vi "HP Loop.vi"(8 "error in (no error)":errorcluster, 11 "ValveControlModule in":refnum<class "ValveControlModule.lvclass">) -> (0 "error out":errorcluster, 3 "ValveControlModule out":refnum<class "ValveControlModule.lvclass">)   [LabVIEW 2020, in "VolatusControl.lvlib" / "ValveControlModule.lvclass"]
uses:
  ValveControlModule.lvclass
  ValveControlModule.lvclass/ValveControlModule.ctl
  <vilib>/Platform/TimedLoop/XDataNode/wakeup.ctl
  <vilib>/Platform/TimedLoop/XDataNode/XDNodeRunTimeDep.lvlib
  <vilib>/Platform/TimedLoop/XDataNode/nitl_modes.ctl
  <vilib>/Platform/TimedLoop/XDataNode/timing_clust.ctl
  <vilib>/platform/TimedLoop/XDataNode/XDataNode.xnode
  Volatus/Module/Module.lvclass
  messages/CmdDigital/Class/Msg.lvclass
  messages/CmdDigital/Data.ctl
  messages/CmdDigital/CmdDigital.lvlib
  messages/CmdDigitalMultiple/Data.ctl
  messages/CmdDigitalMultiple/CmdDigitalMultiple.lvlib
  messages/CmdAnalog/Class/Msg.lvclass
  messages/CmdAnalog/Data.ctl
  messages/CmdAnalog/CmdAnalog.lvlib
  lv-vecto/Vecto/GroupAbstract/GroupAbstract.lvclass
  C:/dev/lv20CE/relink/lv-volatus/Volatus/Module/Module.lvclass
  C:/dev/lv20CE/relink/lv-volatus/VolatusControl/ValveControlModule/ValveControlModule.lvclass
  C:/dev/lv20CE/relink/lv-volatus/messages/CmdDigital/Class/Msg.lvclass
  C:/dev/lv20CE/relink/lv-protoc/LV-Proto/Message/Message.lvclass
  C:/dev/lv20CE/relink/lv-volatus/messages/CmdAnalog/Class/Msg.lvclass
  lv-vecto/Vecto/Group/Group.lvclass
  C:/dev/lv20CE/relink/lv-vecto/Vecto/GroupAbstract/GroupAbstract.lvclass
  C:/dev/lv20CE/relink/lv-vecto/Vecto/Group/Group.lvclass
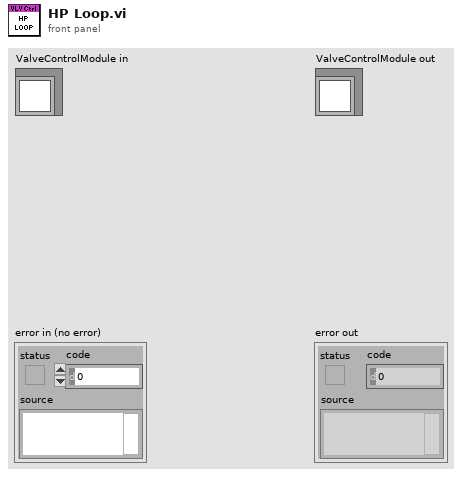
[diagram p1: front panel]
types:
  T1 = typedef "XDNodeRunTimeDep.lvlib/timing_clust.ctl" = cluster{"Expected End [f-1]":u64, "Actual End [f-1]":u64, "Finished Late? [f-1]":bool, "Expected End [i-1]":u64, "Actual End [i-1]":u64, "Finished Late? [i-1]":bool, "Expected Start [i]":u64, "Actual Start [i]":u64, "Expected Start [f]":u64, "Actual Start [f]":u64, "Source Name":string, "Structure Name":string, "Period":i64, "Deadline":i64, "Offset":i64, "Start":i64, "Priority":i32, "Timeout":i32, "Mode":T2, "Wakeup Reason":T3, "Error":errorcluster, "Source Type":string, "Secondary Source Type":string, "Global End Time":u64, "Global Start Time":u64, "Frame Duration":u64, "Iteration Duration":u64, "Assigned CPU":i32, "I/O Scan Engine Mode":u32}
  T2 = typedef "XDNodeRunTimeDep.lvlib/nitl_modes.ctl" = enum32{"No Change", "Process missed periods, maintain original phase", "Discard missed periods, maintain original phase", "Process missed periods, ignore original phase", "Discard missed periods, ignore original phase"}
  T3 = typedef "XDNodeRunTimeDep.lvlib/wakeup.ctl" = enum32{"Normal", "Aborted", "Asynchronous wakeup", "Timing source error", "Timed loop error", "Timeout"}
  T4 = typedef "CmdDigital.lvlib/Data.ctl" = cluster{"channel":string, "value":bool}
  T5 = typedef "CmdDigitalMultiple.lvlib/Data.ctl" = cluster{"values":T4[]}
  T6 = typedef "CmdAnalog.lvlib/Data.ctl" = cluster{"channel":string, "value":dbl}
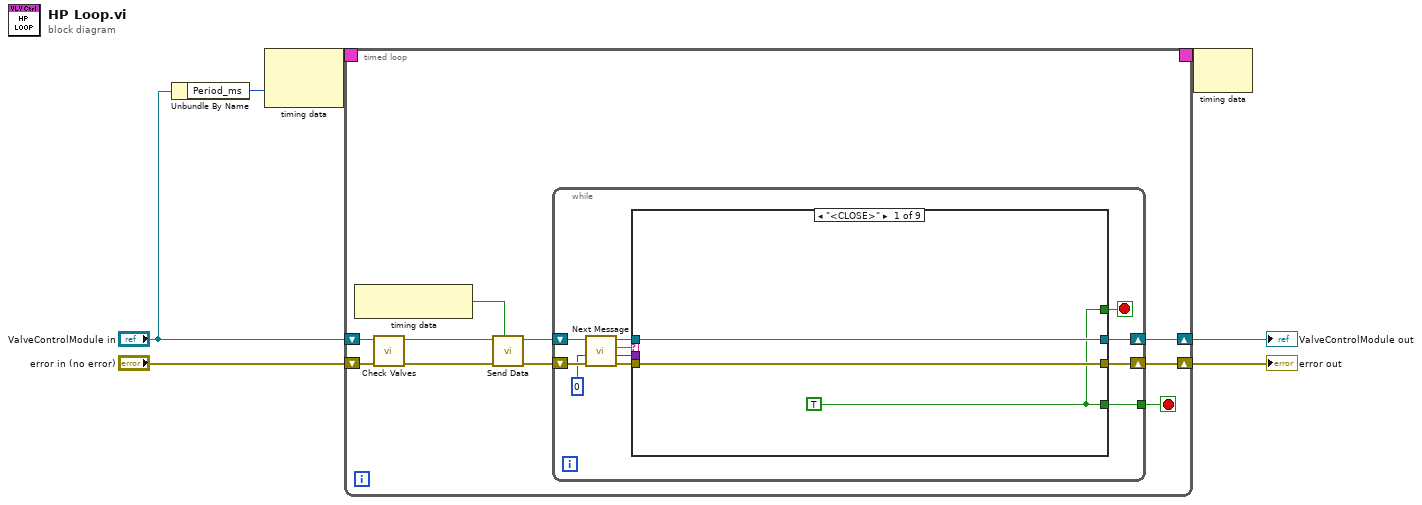
[diagram p0: block diagram]
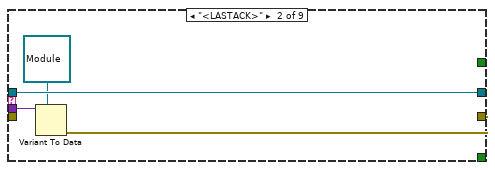
[diagram p2: hidden frame]
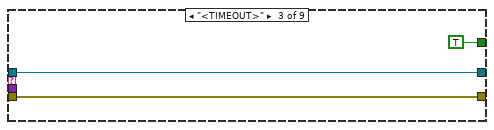
[diagram p3: hidden frame]
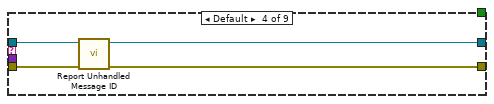
[diagram p4: hidden frame]
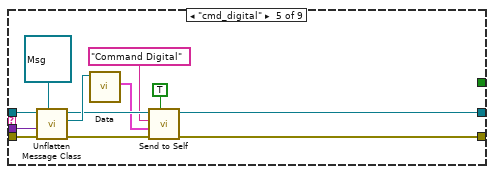
[diagram p5: hidden frame]
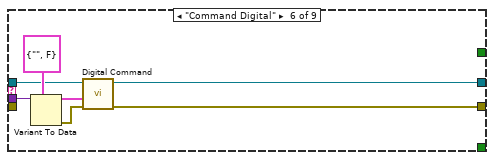
[diagram p6: hidden frame]
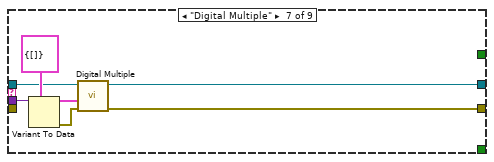
[diagram p7: hidden frame]
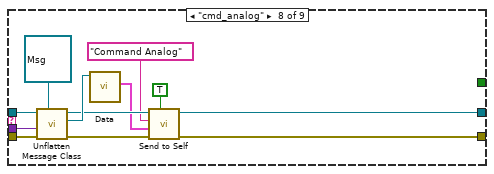
[diagram p8: hidden frame]
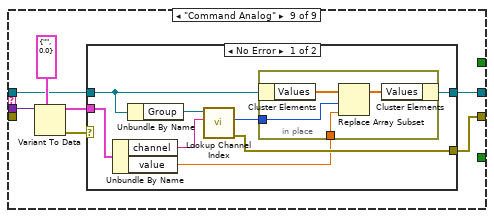
[diagram p9: hidden frame]
diagram:
  n1 = Unbundle By Name("ValveControlModule in") -> ("Period_ms"=w1:i64)
  n2 = node-c288(w1) -> (w7:T1)  [unwired: 1 in]
  n3 = timed-loop {
    shift-right: [w17] -> w4
    shift-left: "ValveControlModule in" -> [w12]
    shift-right: [w16] -> w3
    shift-left: "error in (no error)" -> [w11]
    timing: w7 -> [_]
    timing-out: [_] -> w6
    stop <- w15 stop-if-true
    n4 = node-c288() -> (w8:bool)  [unwired: 1 in]
    n5 = call "Check Valves.vi"("error in (no error)"=w11, "ValveControlModule in"=w12) -> ("error out"=w13:errorcluster, "ValveControlModule out"=w14:refnum<class "ValveControlModule.lvclass">)  [unwired: 8 in]
    n6 = call "Send Data.vi"("Finished Late"=w8, "error in (no error)"=w13, "ValveControlModule in"=w14) -> ("error out"=w10:errorcluster, "ValveControlModule out"=w9:refnum<class "ValveControlModule.lvclass">)  [unwired: 7 in]
    n7 = while {
      tunnel: [w25] -> w15
      shift-right: [w26] -> w16
      shift-left: w10 -> [w23]
      shift-right: [w27] -> w17
      shift-left: w9 -> [w22]
      stop <- w20 stop-if-true
      n8 = call "Next Message.vi"("error in (no error)"=w23, "Timeout ms (-1)"=0, "Module in"=w22) -> ("error out"=w30:errorcluster, "Data"=w24:variant, "ID"=w29:string, "Module out"=w28:refnum<class "ValveControlModule.lvclass">)  [unwired: 5 in]
      n9 = case shown="\"<CLOSE>\"" w29 {
        tunnel: w30 -> [w33 _ w39 w44 w55 _ _ w81 _]
        tunnel: w28 -> [w32 w37 w40 w42 w56 w61 w68 w82 w85]
        tunnel: [w32 w37 w40 w41 w47 w57 w65 w73 w83] -> w27
        tunnel: [w33 w34 w39 w43 w45 w58 w66 w71 w84] -> w26
        tunnel: [w31 _ _ _ _ _ _ _ _] -> w25
        tunnel: w24 -> [_ w36 _ _ w54 w63 w70 w80 w89]
        tunnel: [w31 _ TRUE _ _ _ _ _ _] -> w20
        frame "<CLOSE>" {
          w31 = TRUE
        }
        frame "<LASTACK>" {
          n10 = Variant To Data(type=refnum<class "Module.lvclass"> refnum ("Volatus:Module"), Variant=w36) -> (error out=w34:errorcluster)  [unwired: 1 in, 1 out]
        }
        frame "<TIMEOUT>" {
        }
        frame Default {
          n11 = call "Report Unhandled Message ID.vi"("error in (no error)"=w44, "Module in"=w42) -> ("error out"=w43:errorcluster, "Module out"=w41:refnum<class "ValveControlModule.lvclass">)  [unwired: 8 in]
        }
        frame "cmd_digital" {
          n12 = call "Unflatten Message Class.vi"("Message Type"=refnum<class "Msg.lvclass"> refnum ("CmdDigital.lvlib:Msg.lvclass"), "error in (no error)"=w55, "Data"=w54, "Module in"=w56) -> ("error out"=w50:errorcluster, "Message"=w52:refnum<class "Msg.lvclass">, "Module out"=w51:refnum<class "ValveControlModule.lvclass">)  [unwired: 4 in, 1 out]
          n13 = call "Data.vi"("PB Msg Template in"=w52) -> ("Data"=w48:T4)  [unwired: 8 in, 2 out]
          n14 = call "Send to Self.vi"("High Priority (F)"=TRUE, "error in (no error)"=w50, "Data"=w48, "Message ID"="Command Digital", "Module in"=w51) -> ("error out"=w45:errorcluster, "Module out"=w47:refnum<class "ValveControlModule.lvclass">)  [unwired: 5 in]
        }
        frame "Command Digital" {
          n15 = Variant To Data(type=T4 {"channel"="", "value"=FALSE} ("CmdDigital"), Variant=w63) -> (data=w60:T4, error out=w59:errorcluster)  [unwired: 1 in]
          n16 = call "Digital Command.vi"("error in (no error)"=w59, "CmdDigital"=w60, "ValveControlModule in"=w61) -> ("error out"=w58:errorcluster, "ValveControlModule out"=w57:refnum<class "ValveControlModule.lvclass">)  [unwired: 7 in]
        }
        frame "Digital Multiple" {
          n17 = Variant To Data(type=T5 {"values"=[]} ("CmdDigitalMultiple"), Variant=w70) -> (data=w67:T5, error out=w64:errorcluster)  [unwired: 1 in]
          n18 = call "Digital Multiple.vi"("error in (no error)"=w64, "Data"=w67, "ValveControlModule in"=w68) -> ("error out"=w66:errorcluster, "ValveControlModule out"=w65:refnum<class "ValveControlModule.lvclass">)  [unwired: 7 in]
        }
        frame "cmd_analog" {
          n19 = call "Unflatten Message Class.vi"("Message Type"=refnum<class "Msg.lvclass"> refnum ("CmdAnalog.lvlib:Msg.lvclass"), "error in (no error)"=w81, "Data"=w80, "Module in"=w82) -> ("error out"=w76:errorcluster, "Message"=w78:refnum<class "Msg.lvclass">, "Module out"=w77:refnum<class "ValveControlModule.lvclass">)  [unwired: 4 in, 1 out]
          n20 = call "Data.vi"("PB Msg Template in"=w78) -> ("Data"=w74:T6)  [unwired: 8 in, 2 out]
          n21 = call "Send to Self.vi"("High Priority (F)"=TRUE, "error in (no error)"=w76, "Data"=w74, "Message ID"="Command Analog", "Module in"=w77) -> ("error out"=w71:errorcluster, "Module out"=w73:refnum<class "ValveControlModule.lvclass">)  [unwired: 5 in]
        }
        frame "Command Analog" {
          n22 = Variant To Data(type=T6 {"channel"="", "value"=0.0} ("CmdAnalog"), Variant=w89) -> (data=w86:T6, error out=w87:errorcluster)  [unwired: 1 in]
          n23 = case shown="No Error" w87 {
            selector: w87 -> [_ w103]
            tunnel: w86 -> [w96 _]
            tunnel: w85 -> [w93 w102]
            tunnel: [w97 w103] -> w84
            tunnel: [w90 w102] -> w83
            frame No Error {
              n24 = Unbundle By Name(w96) -> ("channel"=w94:string, "value"=w91:dbl)
              n25 = Unbundle By Name(w93) -> ("Group"=w95:refnum<class "Group.lvclass">)
              n26 = call "Lookup Channel Index.vi"("Channel Name"=w94, "GroupAbstract in"=w95) -> ("error out"=w97:errorcluster, "Index"=w92:i32)  [unwired: 7 in, 1 out]
              n27 = in-place {
                in-place-border: w92 -> [w100]
                in-place-border: w91 -> [w99]
                n28 = in-place-cluster #1(w93) -> ("Values"=w101:dbl[])
                n29 = Replace Array Subset(array=w101, new element=w99, index=w100) -> (w98:dbl[])
                n30 = in-place-cluster #1("Values"=w98) -> (w90:refnum<class "ValveControlModule.lvclass">)
              }
            }
            frame Error {
            }
          }
        }
      }
    }
  }
  "error out" <- w3
  "ValveControlModule out" <- w4
  n31 = node-c288(w6) -> ()  [unwired: 1 out]
